vi "Exec IO.vi"() -> ()   [LabVIEW 2023]
uses:
  <vilib>/eio/EIONode/EIONode.xnode
  <vilib>/Platform/TimedLoop/XDataNode/wakeup.ctl
  <vilib>/Platform/TimedLoop/XDataNode/XDNodeRunTimeDep.lvlib
  <vilib>/Platform/TimedLoop/XDataNode/nitl_modes.ctl
  <vilib>/Platform/TimedLoop/XDataNode/timing_clust.ctl
  <vilib>/platform/TimedLoop/XDataNode/XDataNode.xnode
  Front Panel Globals.vi
  <vilib>/rvi/eio/common/nirviEmuTemplateMethod_errors.vi
panel:
  out "Voltage Data":sgl[](array[numeric])
  out "Voltage Looprate":sgl
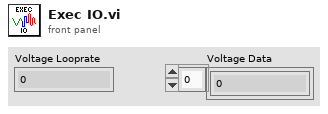
[diagram p1: front panel]
types:
  T1 = typedef "XDNodeRunTimeDep.lvlib/timing_clust.ctl" = cluster{"Expected End [f-1]":u64, "Actual End [f-1]":u64, "Finished Late? [f-1]":bool, "Expected End [i-1]":u64, "Actual End [i-1]":u64, "Finished Late? [i-1]":bool, "Expected Start [i]":u64, "Actual Start [i]":u64, "Expected Start [f]":u64, "Actual Start [f]":u64, "Source Name":string, "Structure Name":string, "Period":i64, "Deadline":i64, "Offset":i64, "Start":i64, "Priority":i32, "Timeout":i32, "Mode":T2, "Wakeup Reason":T3, "Error":errorcluster, "Source Type":string, "Secondary Source Type":string, "Global End Time":u64, "Global Start Time":u64, "Frame Duration":u64, "Iteration Duration":u64, "Assigned CPU":i32, "I/O Scan Engine Mode":u32}
  T2 = typedef "XDNodeRunTimeDep.lvlib/nitl_modes.ctl" = enum32{"No Change", "Process missed periods, maintain original phase", "Discard missed periods, maintain original phase", "Process missed periods, ignore original phase", "Discard missed periods, ignore original phase"}
  T3 = typedef "XDNodeRunTimeDep.lvlib/wakeup.ctl" = enum32{"Normal", "Aborted", "Asynchronous wakeup", "Timing source error", "Timed loop error", "Timeout"}
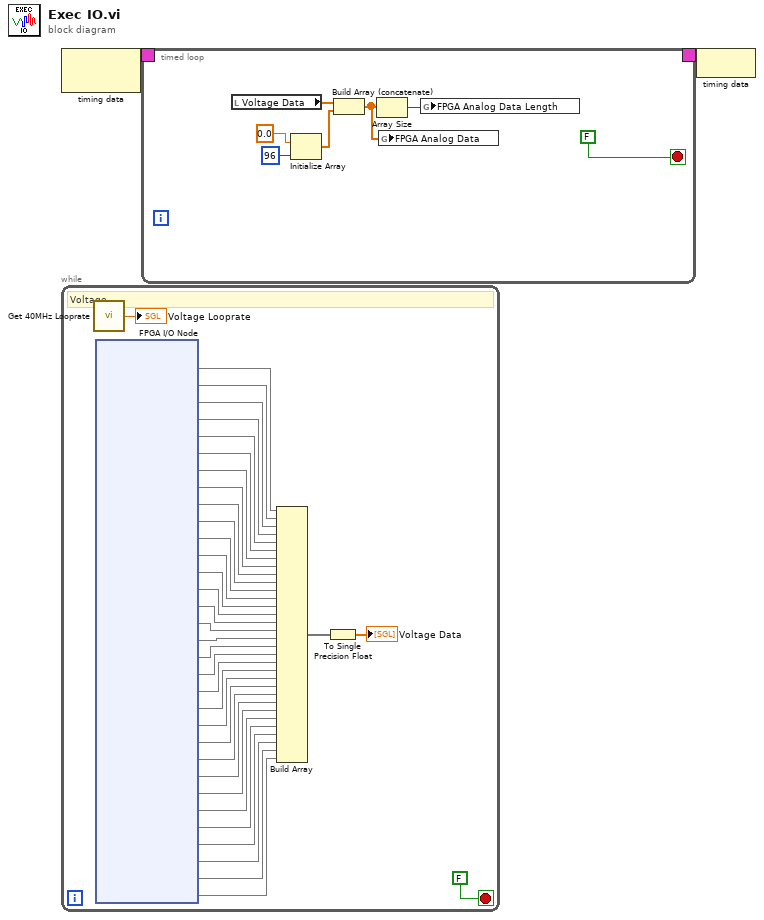
[diagram p0: block diagram]
diagram:
  n1 = node-c288() -> (w2:T1)  [unwired: 1 in]
  n2 = while {
    stop <- FALSE stop-if-true
    # "Voltage"
    n3 = call "Get 40MHz Looprate.vi"() -> ("Looprate"=→"Voltage Looprate":sgl)  [unwired: 5 in]
    n4 = xnode "FPGA I/O Node"() -> ("Mod3/AI0"=w35, "Mod3/AI1"=w34, "Mod3/AI2"=w33, "Mod3/AI3"=w32, "Mod3/AI4"=w31, "Mod3/AI5"=w30, "Mod3/AI6"=w29, "Mod3/AI7"=w28, "Mod3/AI16"=w27, "Mod3/AI17"=w25, "Mod3/AI18"=w24, "Mod3/AI19"=w23, "Mod3/AI20"=w22, "Mod3/AI21"=w21, "Mod3/AI22"=w20, "Mod3/AI23"=w19, "Mod6/AI0"=w18, "Mod6/AI1"=w17, "Mod6/AI2"=w16, "Mod6/AI3"=w15, "Mod6/AI4"=w14, "Mod6/AI5"=w13, "Mod6/AI6"=w12, "Mod6/AI7"=w11, "Mod6/AI16"=w10, "Mod6/AI17"=w9, "Mod6/AI18"=w8, "Mod6/AI19"=w7, "Mod6/AI20"=w6, "Mod6/AI21"=w5, "Mod6/AI22"=w4, "Mod6/AI23"=w3)  [unwired: 32 in, 32 out]
    n5 = Build Array(w35, w34, w33, w32, w31, w30, w29, w28, w27, w25, w24, w23, w22, w21, w20, w19, w18, w17, w16, w15, w14, w13, w12, w11, w10, w9, w8, w7, w6, w5, w4, w3) -> (w26:void[])
    n6 = To Single Precision Float(number=w26) -> (single precision float=→"Voltage Data":sgl[])
  }
  n7 = timed-loop {
    timing: w2 -> [_]
    timing-out: [_] -> w1
    stop <- FALSE stop-if-true
    n8 = local read "Voltage Data"() -> (w39:sgl[])
    n9 = Initialize Array(sgl 0.0 ("element"), 96 ("dimension size")) -> (w41:sgl[])
    n10 = Build Array (concatenate)(w39, w41) -> (w44:sgl[])
    n11 = Array Size(array=w44) -> (size(s)=w40:i32)
    n12 = global write "Front Panel Globals.vi" "FPGA Analog Data"(w44) -> ()
    n13 = global write "Front Panel Globals.vi" "FPGA Analog Data Length"(w40) -> ()
  }
  n14 = node-c288(w1) -> ()
